vi "AutoGoHome.vi"(8 "error in (no error)":errorcluster) -> (0 "error out":errorcluster)   [LabVIEW 2023]
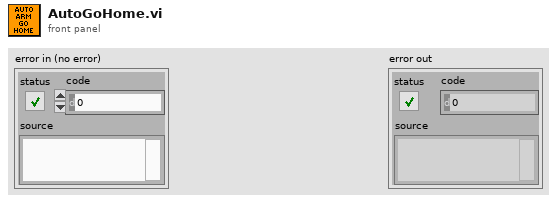
[diagram p1: front panel]
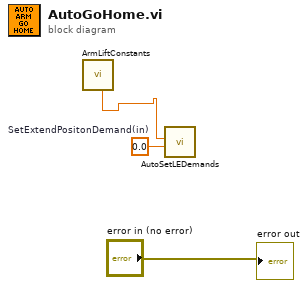
[diagram p0: block diagram]
diagram:
  w3 = 0.0  # SetExtendPositonDemand(in)
  n1 = call "ArmLiftConstants.vi"() -> ("Default Angle"=w1:dbl)  [unwired: 8 in, 3 out]
  n2 = call "AutoSetLEDemands.vi"("SetExtendPositonDemand(in)"=w3, "SetLIftPostionDemand(d)"=w1) -> ()  [unwired: 9 in, 1 out]
  "error out" <- "error in (no error)"
